vi "Copy Inline to Async.vi"(8 "error in (no error)":errorcluster, 11 "Buffers in":refnum<class "Buffers.lvclass">) -> (0 "error out":errorcluster, 3 "Buffers out":refnum<class "Buffers.lvclass">)   [LabVIEW 2017, in "DSF Core.lvlib" / "Buffers.lvclass"]
uses:
  Buffers.lvclass
  Buffers.lvclass/Buffers.ctl
  Buffer/Buffer.lvclass
  C:/Git/DSF/LabVIEW-Memory/Source/Classes/Pointer/Pointer.lvclass
  LabVIEW-Memory/Source/Classes/Pointer/Pointer.lvclass
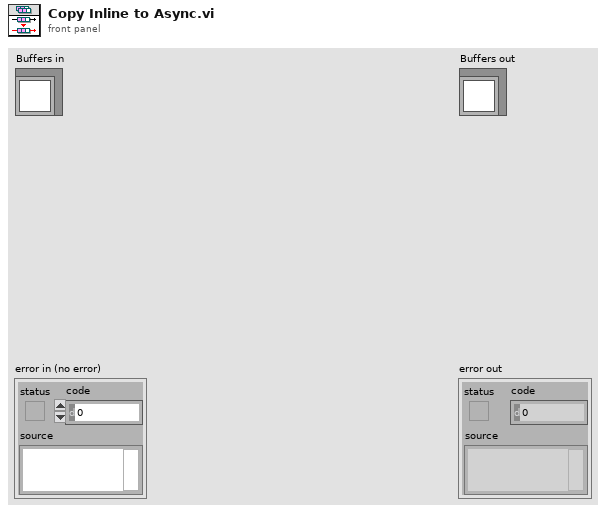
[diagram p1: front panel]
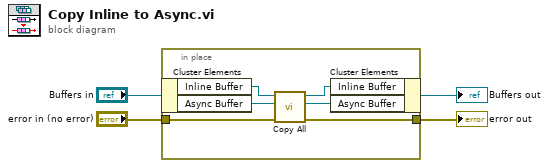
[diagram p0: block diagram]
diagram:
  n1 = in-place {
    in-place-border: "error in (no error)" -> [w8]
    in-place-border: [w7] -> w2
    n2 = in-place-cluster #1("Buffers in") -> ("Inline Buffer"=w9:refnum<class "Buffer.lvclass">, "Async Buffer"=w10:refnum<class "Buffer.lvclass">)
    n3 = call "Copy All.vi"("error in (no error)"=w8, "dst Pointer in"=w10, "src Pointer in"=w9) -> ("error out"=w7:errorcluster, "dst Pointer out"=w6:refnum<class "Buffer.lvclass">, "src Pointer out"=w5:refnum<class "Buffer.lvclass">)  [unwired: 6 in]
    n4 = in-place-cluster #1("Inline Buffer"=w5, "Async Buffer"=w6) -> (→"Buffers out":refnum<class "Buffers.lvclass">)
  }
  "error out" <- w2
